vi "TestSeqGenerator.vi"() -> ()   [LabVIEW 2019]
uses:
  GUIHandler/GUI_Handler_Seq.lvclass
  testSeq/TestSeqClass.lvclass
panel:
  out "ResultListBox 3":i32(listbox)=-1
  in  "ResultListBox 2":i32(listbox)=-1
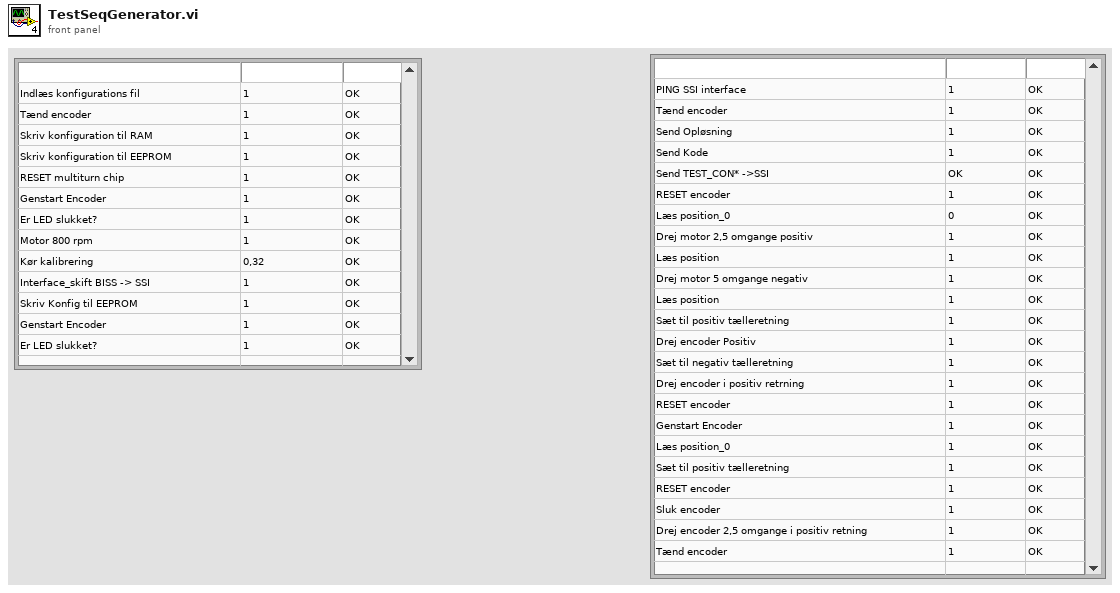
[diagram p1: front panel]
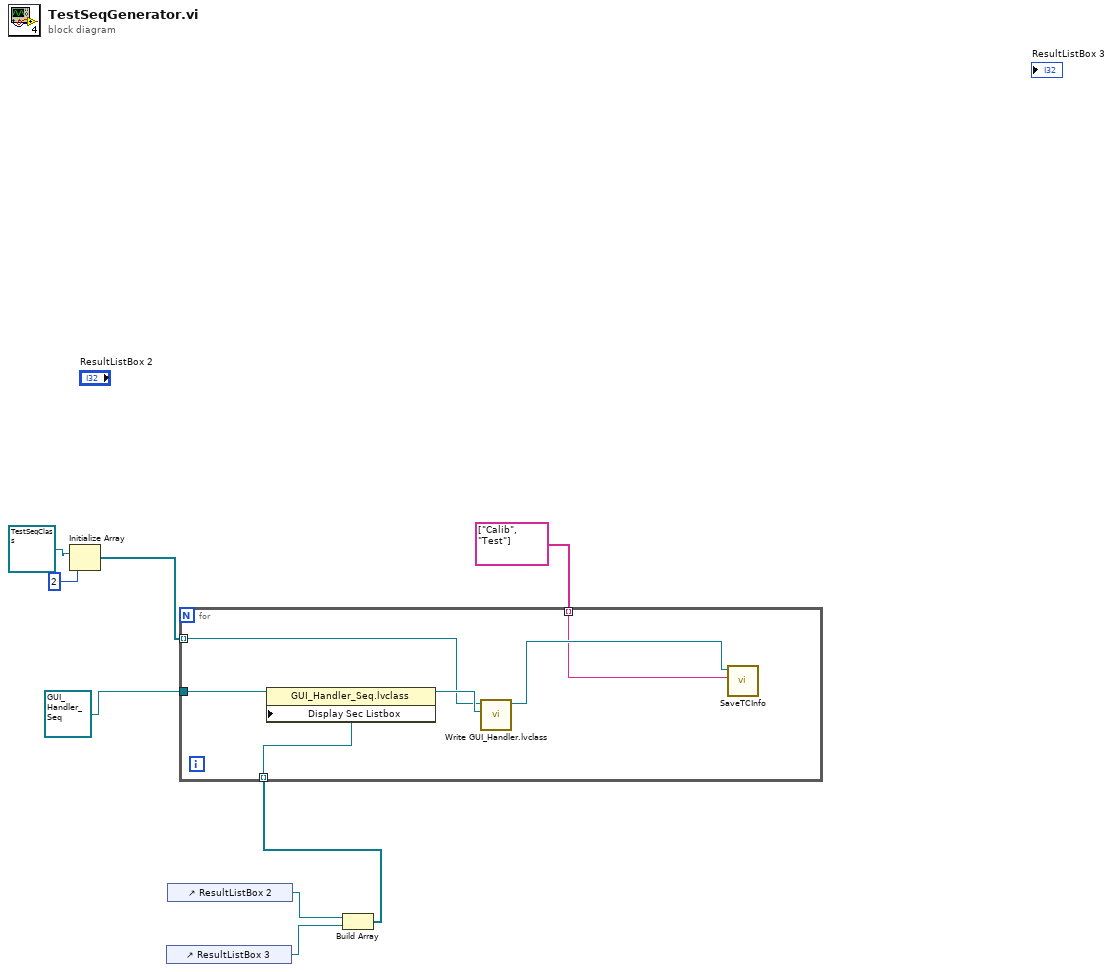
[diagram p0: block diagram]
diagram:
  n1 = Initialize Array(refnum<class "TestSeqClass.lvclass"> refnum ("TestSeqClass.lvclass"), 2 ("dimension size")) -> (w1:refnum<class "TestSeqClass.lvclass">[])
  n2 = control-ref of="ResultListBox 3"() -> (w5:refnum<vi>)
  n3 = control-ref of="ResultListBox 2"() -> (w6:refnum<vi>)
  n4 = Build Array(w6, w5) -> (w4:refnum<vi>[])
  n5 = for {
    tunnel: string[] ["Calib", "Test"] -> [w9] mode=indexing
    tunnel: refnum<class "GUI_Handler_Seq.lvclass"> refnum ("GUI_Handler.lvclass") -> [w13]
    tunnel: w4 -> [w12] mode=indexing
    tunnel: w1 -> [w11] mode=indexing
    n6 = property class="GUI_Handler_Seq.lvclass"(reference=w13, "Display Sec Listbox"=w12) -> (reference out=w14:refnum<class "GUI_Handler_Seq.lvclass">)  [unwired: 1 in, 1 out]
    n7 = call-dynamic "Write GUI_Handler.lvclass.vi"("GUI_Handler.lvclass"=w14, "TestSeqClass in"=w11) -> ("TestSeqClass out"=w10:refnum<class "TestSeqClass.lvclass">)  [unwired: 8 in, 1 out]
    n8 = call "SaveTCInfo.vi"("TestType"=w9, "TestSeqClass.lvclass"=w10) -> ()  [unwired: 8 in, 2 out]
  }
